vi "init.vi"(6 "Comms":string(combo)="330", 7 "Timeout Value (ms)":u32=5000, 8 "error in (no error)":errorcluster, 10 "Load default parameters?":bool, 11 "VISA resource name":refnum<visa-resource-name>) -> (0 "error out":errorcluster, 3 "VISA resource name out":refnum<visa-resource-name>)   [LabVIEW 2018]
doc: "Start the active process or continue a process that is in the STOP state."
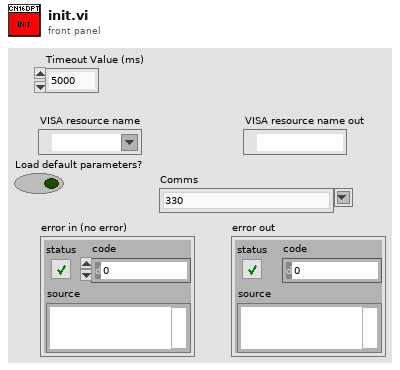
[diagram p1: front panel]
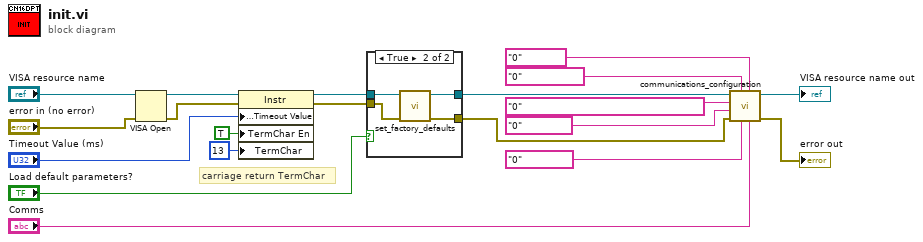
[diagram p0: block diagram]
diagram:
  # "carriage return TermChar"
  n1 = VISA Open(error in (no error)="error in (no error)", VISA resource name="VISA resource name") -> (VISA resource name=w17:refnum<visa-resource-name>, error out=w15:errorcluster)  [unwired: 3 in]
  n2 = property class="Instr"(reference=w17, error in=w15, "General Settings:Timeout Value"="Timeout Value (ms)", "TermChar En"=TRUE ("Message Based Settings:Termination Character Enable"), "TermChar"=u8 13 ("Message Based Settings:Termination Character")) -> (reference out=w12:refnum<visa-resource-name>, error out=w11:errorcluster)
  n3 = case shown="True" "Load default parameters?" {
    tunnel: w12 -> [w21 w26]
    tunnel: w11 -> [w22 w24]
    tunnel: [w21 w25] -> w4
    tunnel: [w22 w23] -> w3
    frame False {
    }
    frame True {
      n4 = call "set_factory_defaults.vi"("error in (no error)"=w24, "VISA Refnum in"=w26) -> ("error out"=w23:errorcluster, "VISA Refnum out"=w25:refnum<visa-resource-name>)  [unwired: 8 in]
    }
  }
  n5 = call "communications_configuration.vi"("Comms"="Comms", "Protocol"="0", "Separation char (Omega protocol, continuous data mode)"="0", "Data mode"="0", "error in (no error)"=w3, "Response echo enabled"="0", "Line feed enabled"="0", "VISA Refnum in"=w4) -> ("error out"=→"error out":errorcluster, "VISA Refnum out"=→"VISA resource name out":refnum<visa-resource-name>)  [unwired: 2 in]
